vi "Vi_ConnectionCarte.vi"() -> (2 "Deverouillé":bool, 3 "Connecté":bool)   [LabVIEW 2015]
uses:
  <userlib>/ICNC/ICNC2.lvlib
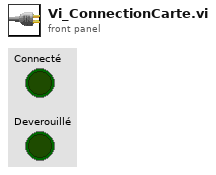
[diagram p1: front panel]
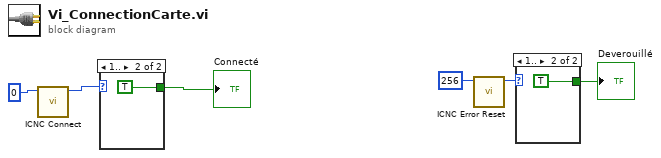
[diagram p0: block diagram]
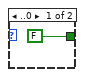
[diagram p2: hidden frame]
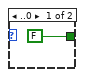
[diagram p3: hidden frame]
diagram:
  n1 = call <userlib>:"ICNC Connect.vi"("ICNC_Number"=0) -> ("function return"=w4:u32)  [unwired: 9 in, 1 out]
  n2 = case shown="1.." w4 {
    tunnel: [FALSE TRUE] -> w1
    frame ..0 {
    }
    frame 1.. {
    }
  }
  "Connecté" <- w1
  n3 = call <userlib>:"ICNC Error Reset.vi"("ErrorBits"=256) -> ("function return"=w5:u32)  [unwired: 9 in, 1 out]
  n4 = case shown="1.." w5 {
    tunnel: [FALSE TRUE] -> w2
    frame ..0 {
    }
    frame 1.. {
    }
  }
  "Deverouillé" <- w2
